vi "Pause.vi"(8 "error in (no error)":errorcluster, 11 "EPOS4 Settings in":T1={"VISA resource name"="", "axis"={"keyHandle"=0, "nodeId"=1}, "Simulated?"=FALSE}) -> (0 "error out":errorcluster, 1 "Connection Error":bool, 3 "EPOS4 Settings out":T1={"VISA resource name"="", "axis"={"keyHandle"=0, "nodeId"=1}, "Simulated?"=FALSE})   [LabVIEW 2018, in "EPOS4.lvlib"]
uses:
  EPOS4.lvlib
  Controls/EPOS Communication Settings.ctl
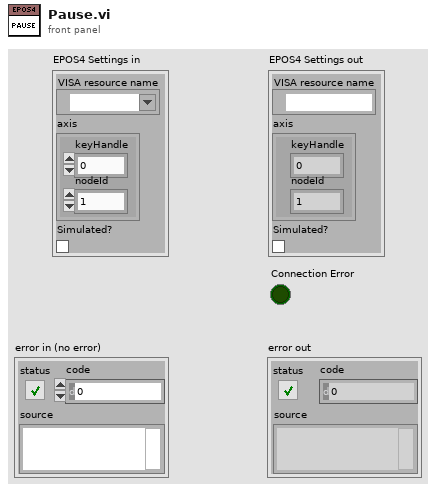
[diagram p1: front panel]
types:
  T1 = typedef "EPOS4.lvlib/EPOS Communication Settings.ctl" = cluster{"VISA resource name":refnum<visa-resource-name>, "axis":cluster{"keyHandle":u32, "nodeId":u16}, "Simulated?":bool}
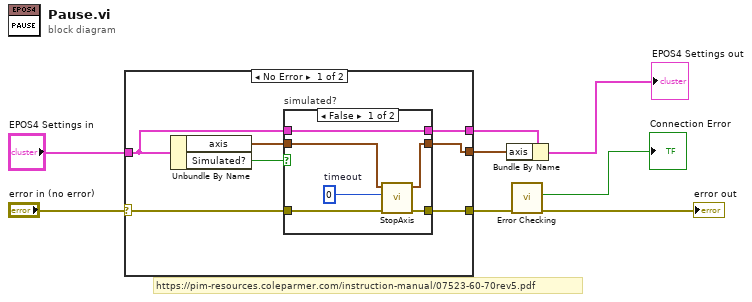
[diagram p0: block diagram]
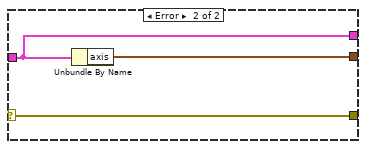
[diagram p3: hidden frame]
diagram:
  # "https://pim-resources.coleparmer.com/instruction-manual/07523-60-70rev5.pdf"
  n1 = case shown="No Error" "error in (no error)" {
    selector: "error in (no error)" -> [w13 w27]
    tunnel: [w9 w26] -> w3
    tunnel: "EPOS4 Settings in" -> [w10 w26]
    tunnel: [w12 w25] -> w2
    tunnel: [w11 w27] -> w8
    frame No Error {
      n2 = Unbundle By Name(w10) -> ("axis"=w15:cluster{"keyHandle":u32, "nodeId":u16}, "Simulated?"=w14:bool)
      n3 = case "simulated?" shown="False" w14 {
        tunnel: [w18 w24] -> w12
        tunnel: w15 -> [w20 w24]
        tunnel: w13 -> [w19 w23]
        tunnel: [w16 w23] -> w11
        tunnel: w10 -> [w17 w22]
        tunnel: [w17 w22] -> w9
        frame False {
          w21 = u32 0  # timeout
          n4 = call "StopAxis.vi"("error in (no error)"=w19, "timeout"=w21, "axis in"=w20) -> ("error out"=w16:errorcluster, "axis out"=w18:cluster{"keyHandle":u32, "nodeId":u16})  [unwired: 3 in]
        }
        frame True {
        }
      }
    }
    frame Error {
      n5 = Unbundle By Name(w26) -> ("axis"=w25:cluster{"keyHandle":u32, "nodeId":u16})
    }
  }
  n6 = Bundle By Name(cluster=w3, "axis"=w2) -> (→"EPOS4 Settings out":T1)
  n7 = call "Error Checking.vi"("error in (no error)"=w8) -> ("error out"=→"error out":errorcluster, "Connection Error"=→"Connection Error":bool)  [unwired: 8 in, 1 out]
